vi "AddError__slk_mt.vi"(8 "error in (no error)":errorcluster, 10 "vi name":string, 11 "application reference":refnum<vi>) -> (0 "error out":errorcluster)   [LabVIEW 2013, in "Lazyboots Menu Tool.lvlib"]
doc: "This VI is the core of <b>Add Error</b> function, and will be called by corresponding menu launcher."
uses:
  Library/Lazyboots Menu Tool.lvlib
  <vilib>/Utility/config.llb/NI_LVConfig.lvlib
  Private/AddError/TypeDef/TypeDef_AddErrorState__slk_mt.ctl
  <vilib>/Utility/miscctls.llb/LVPositionTypeDef.ctl
panel:
  # "AddError__slk_mt.vi\nThis VI is the core of <b>Add Error</b> function, and will be called by corresponding menu launcher.\n\nNOTICE -- YOU MUST LEAVE THIS NOTICE IN PLACE.\n\nCopyright (c) 2011, LIANG LIU Shawn.Liu.cn@gmail.com\nAll rights reserved.\n\nRedistribution and use in source and binary forms, with or without modification, are permitted provided that the following conditions are met:\n-Redistributions of source code must retain the above copyright notice, this list of conditions and the following disclaimer.\n-Redistributions in binary form must reproduce the above copyright notice, this list of conditions and the following disclaimer in the documentation and/or other materials provided with the distribution.\n-Neither the name of the eLp nor the names of its contributors may be used to endorse or promote products derived from this software without specific prior written permission.\n\nTHIS SOFTWARE IS PROVIDED BY THE COPYRIGHT HOLDERS AND CONTRIBUTORS \"AS IS\" AND ANY EXPRESS OR IMPLIED WARRANTIES, INCLUDING, BUT NOT LIMITED TO, THE IMPLIED WARRANTIES OF MERCHANTABILITY AND FITNESS FOR A PARTICULAR PURPOSE ARE DISCLAIMED. IN NO EVENT SHALL THE COPYRIGHT HOLDER OR CONTRIBUTORS BE LIABLE FOR ANY DIRECT, INDIRECT, INCIDENTAL, SPECIAL, EXEMPLARY, OR CONSEQUENTIAL DAMAGES (INCLUDING, BUT NOT LIMITED TO, PROCUREMENT OF SUBSTITUTE GOODS OR SERVICES; LOSS OF USE, DATA, OR PROFITS; OR BUSINESS INTERRUPTION) HOWEVER CAUSED AND ON ANY THEORY OF LIABILITY, WHETHER IN CONTRACT, STRICT LIABILITY, OR TORT (INCLUDING NEGLIGENCE OR OTHERWISE) ARISING IN ANY WAY OUT OF THE USE OF THIS SOFTWARE, EVEN IF ADVISED OF THE POSSIBILITY OF SUCH DAMAGE."
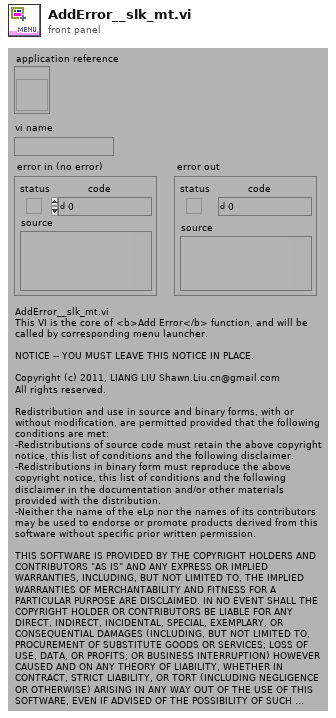
[diagram p1: front panel]
types:
  T1 = typedef "LVPositionTypeDef.ctl" = cluster{"Left":i32, "Top":i32}
  T2 = typedef "Lazyboots Menu Tool.lvlib/TypeDef_AddErrorState__slk_mt.ctl" = enum16{"Read Configure", "Get Menu Launch VI", "Get GObject Rectangle", "Calculate Error In Left Position", "Calculate Error In Top Position", "Undo.Start", "Add Error In", "Calculate Error Out Left Position", "Add Error Out", "Wire to Connector?", "Wire to Connector", "Undo.End/Fail", "End"}
  T3 = typedef "NI_LVConfig.lvlib/Config Data RefNum.ctl" = refnum<k1>
  T4 = typedef "Lazyboots Menu Tool.lvlib/TypeDef_AddErrorConfigure__slk_mt.ctl" = cluster{"Frame Width":u32, "Snap to Grid":bool, "FP Grid Size":u32, "Wire to Connector":bool, "Connector Pattern":u32, "Control Style":string, "Error Style":string}
  T5 = typedef "LVPointTypeDef.ctl" = cluster{"Horizontal":i16, "Vertical":i16}
  T6 = cluster{"left":i16, "top":i16, "right":i16, "bottom":i16}
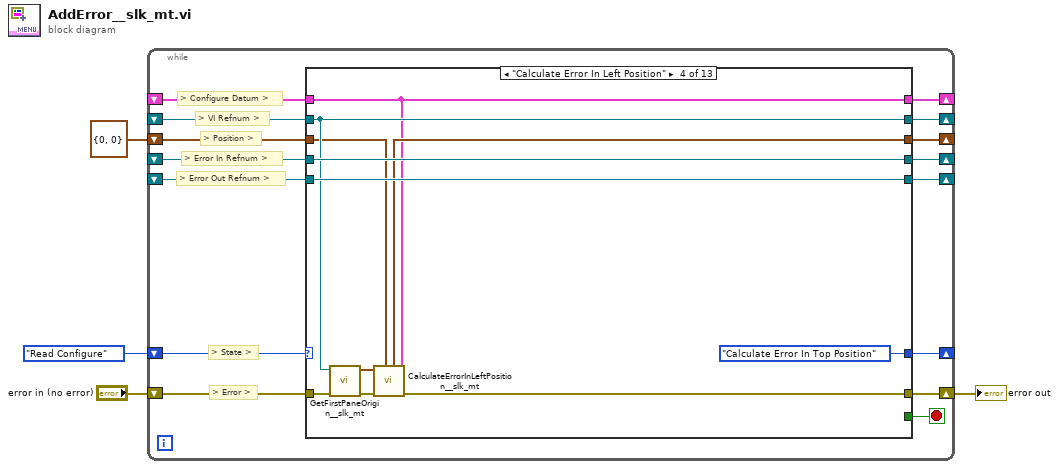
[diagram p0: block diagram]
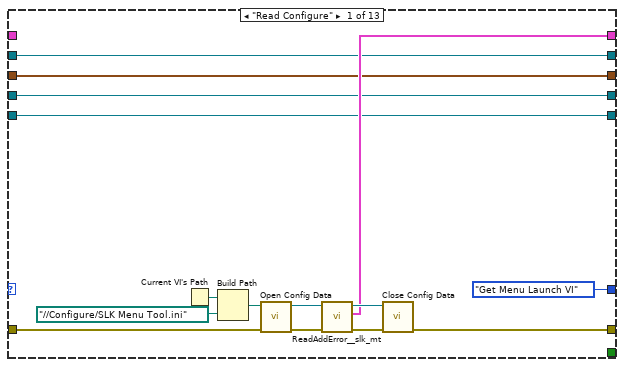
[diagram p2: hidden frame]
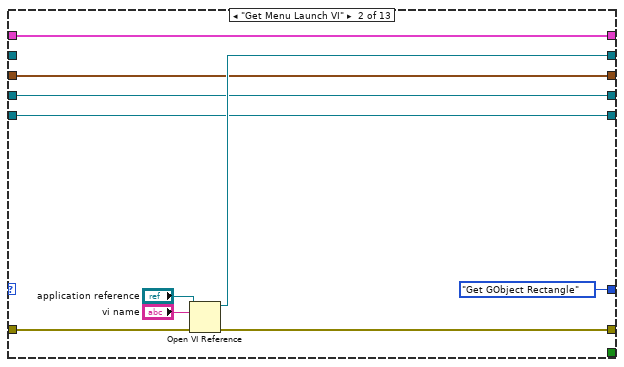
[diagram p3: hidden frame]
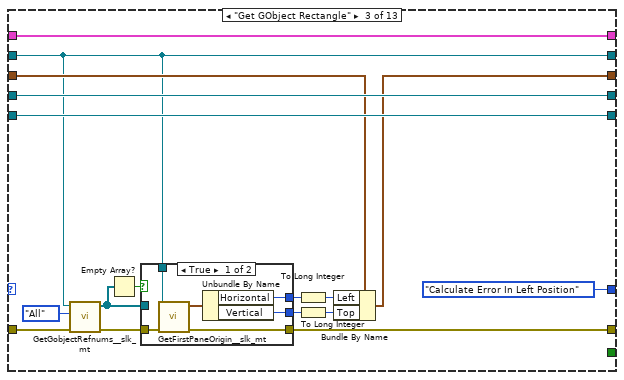
[diagram p4: hidden frame]
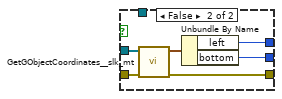
[diagram p5: hidden frame]
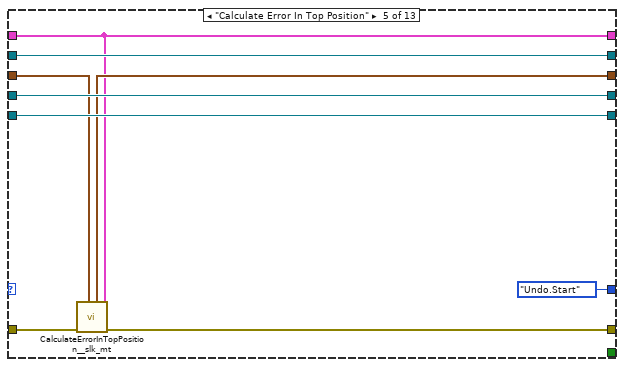
[diagram p6: hidden frame]
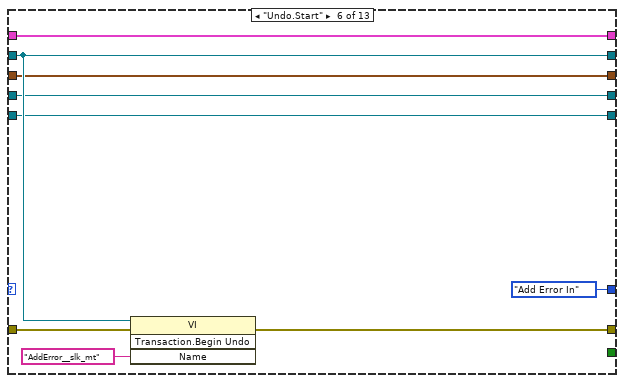
[diagram p7: hidden frame]
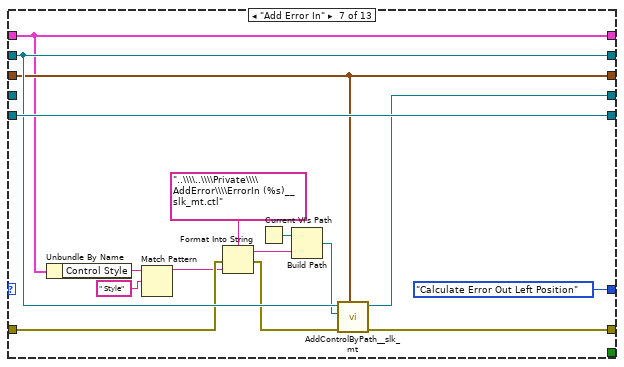
[diagram p8: hidden frame]
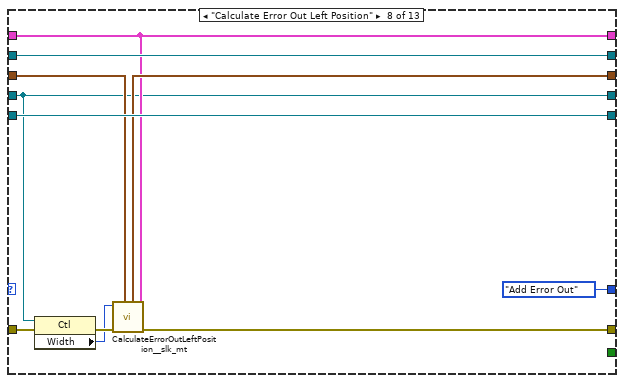
[diagram p9: hidden frame]
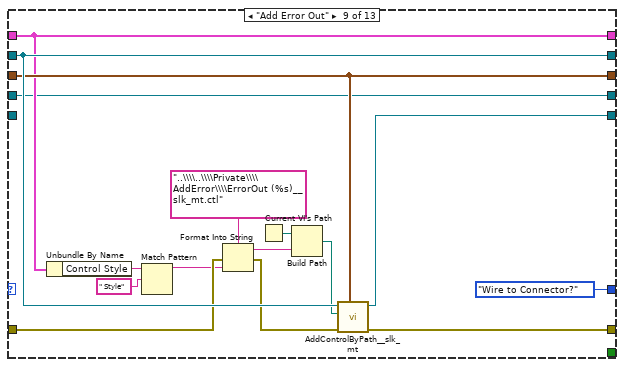
[diagram p10: hidden frame]
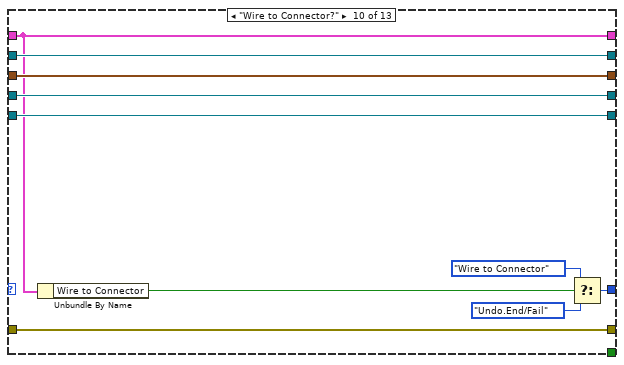
[diagram p11: hidden frame]
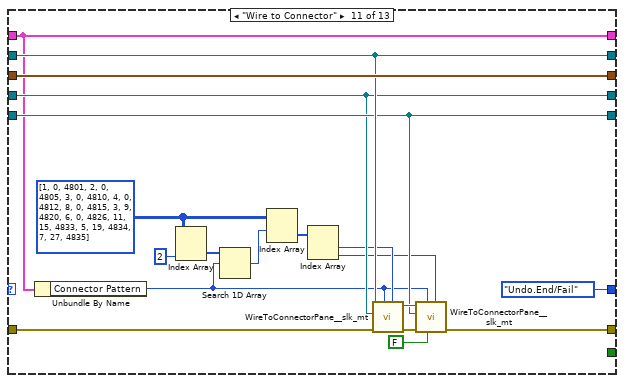
[diagram p12: hidden frame]
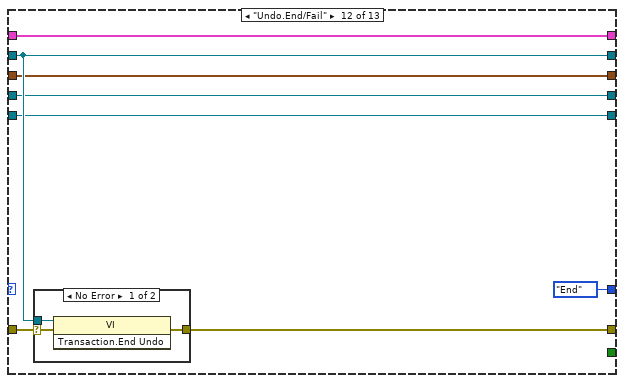
[diagram p13: hidden frame]
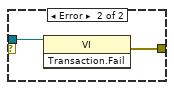
[diagram p14: hidden frame]
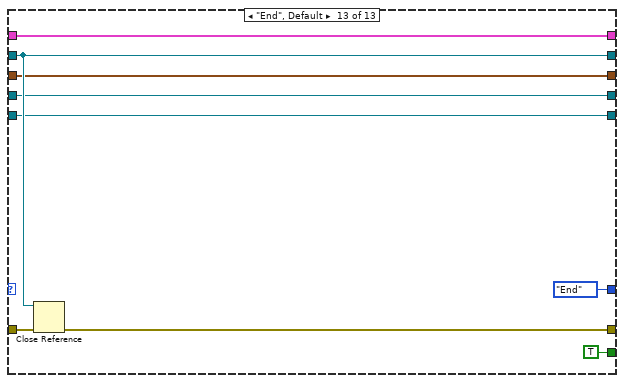
[diagram p15: hidden frame]
diagram:
  n1 = while {
    shift-right: [w16] -> _
    shift-left: TypeDef_AddErrorState__slk_mt."Read Configure" ("State") -> [w19]
    shift-right: [w17] -> w1
    shift-left: "error in (no error)" -> [w18]
    shift-right: [w14] -> _
    shift-left: _ -> [w15]
    shift-right: [w12] -> _
    shift-left: _ -> [w13]
    shift-right: [w7] -> _
    shift-left: T1 {"Left"=0, "Top"=0} ("Position") -> [w10]
    shift-right: [w6] -> _
    shift-left: _ -> [w9]
    shift-right: [w5] -> _
    shift-left: _ -> [w8]
    stop <- w11 stop-if-true
    # "> Error Out Refnum >"
    # "> Error In Refnum >"
    # "> Position >"
    # "> VI Refnum >"
    # "> Configure Datum >"
    # "> Error >"
    # "> State >"
    n2 = case shown="\"Calculate Error In Left Position\"" w19 {
      tunnel: w18 -> [w28 w44 w60 w82 w85 w101 w106 w122 w133 w155 w167 w180 w191]
      tunnel: [w26 w42 w56 w81 w91 w100 w116 w128 w144 w155 w166 w179 w193] -> w17
      tunnel: [TypeDef_AddErrorState__slk_mt."Get Menu Launch VI" ("State") TypeDef_AddErrorState__slk_mt."Get GObject Rectangle" ("State") TypeDef_AddErrorState__slk_mt."Calculate Error In Left Position" ("State") TypeDef_AddErrorState__slk_mt."Calculate Error In Top Position" ("State") TypeDef_AddErrorState__slk_mt."Undo.Start" ("State") TypeDef_AddErrorState__slk_mt."Add Error In" ("State") TypeDef_AddErrorState__slk_mt."Calculate Error Out Left Position" ("State") TypeDef_AddErrorState__slk_mt."Add Error Out" ("State") TypeDef_AddErrorState__slk_mt."Wire to Connector?" ("State") w152 TypeDef_AddErrorState__slk_mt."Undo.End/Fail" ("State") TypeDef_AddErrorState__slk_mt."End" ("State") TypeDef_AddErrorState__slk_mt."End" ("State")] -> w16
      tunnel: w15 -> [_ w41 w61 w75 w87 w102 w112 w124 w141 w147 w164 w182 w196]
      tunnel: [w24 w41 w61 w75 w87 w102 w112 w124 w141 w147 w164 w182 w196] -> w14
      tunnel: w13 -> [w23 _ w45 w79 w90 w99 w115 w127 w143 w151 w172 w178 w192]
      tunnel: [w23 w40 w45 w79 w90 w99 w115 w127 w143 w151 w172 w178 w192] -> w12
      tunnel: [_ _ _ _ _ _ _ _ _ _ _ _ TRUE] -> w11
      tunnel: w10 -> [w22 w38 w50 w77 w89 w96 w114 w126 w142 w150 w174 w177 w190]
      tunnel: w9 -> [w21 w37 w52 w84 w93 w95 _ w120 w135 w149 w169 w176 w189]
      tunnel: w8 -> [w20 w36 w51 w83 w92 w94 w117 w129 _ w148 w170 w175 w188]
      tunnel: [w22 w38 w49 w76 w88 w96 w114 w125 w142 w150 w174 w177 w190] -> w7
      tunnel: [w21 w37 w52 w84 w93 w95 w113 w120 w135 w149 w169 w176 w189] -> w6
      tunnel: [w20 w36 w51 w83 w92 w94 w117 w129 w134 w148 w170 w175 w188] -> w5
      frame "Read Configure" {
        n3 = Current VI's Path() -> (path=w30:path)
        n4 = Build Path(base path=w30, name or relative path=path "../../Configure/SLK Menu Tool.ini") -> (appended path=w29:path)
        n5 = call <vilib>:"Open Config Data.vi"("error in (no error)"=w28, "configuration file path"=w29) -> ("error out"=w33:errorcluster, "refnum"=w34:T3)  [unwired: 7 in, 1 out]
        n6 = call "ReadAddError__slk_mt.vi"("error in (no error)"=w33, "refnum in"=w34) -> ("error out"=w32:errorcluster, "add error configure"=w24:T4, "refnum out"=w31:T3)  [unwired: 7 in]
        n7 = call <vilib>:"Close Config Data.vi"("error in (no error)"=w32, "refnum"=w31) -> ("error out"=w26:errorcluster)  [unwired: 8 in, 1 out]
      }
      frame "Get Menu Launch VI" {
        n8 = Open VI Reference(application reference (local)="application reference", vi path="vi name", error in (no error)=w44) -> (vi reference=w40:refnum<vi>, error out=w42:errorcluster)  [unwired: 3 out]
      }
      frame "Get GObject Rectangle" {
        n9 = call "GetGobjectRefnums__slk_mt.vi"("error in (no error)"=w60, "from (Selected)"=enum16{"All", "Selected"}."All", "vi refnum in"=w45) -> ("error out"=w59:errorcluster, "generic objects refnums out"=w57:refnum<vi>[])  [unwired: 7 in]
        n10 = Empty Array?(array=w57) -> (empty?=w46:bool)
        n11 = case shown="True" w46 {
          tunnel: w59 -> [w67 w73]
          tunnel: w57 -> [_ w72]
          tunnel: [w66 w71] -> w56
          tunnel: [w64 w69] -> w54
          tunnel: [w63 w68] -> w53
          tunnel: w45 -> [w62 _]
          frame True {
            n12 = call "GetFirstPaneOrigin__slk_mt.vi"("error in (no error)"=w67, "vi refnum in"=w62) -> ("error out"=w66:errorcluster, "origin"=w65:T5)  [unwired: 8 in]
            n13 = Unbundle By Name(w65) -> ("Horizontal"=w64:i16, "Vertical"=w63:i16)
          }
          frame False {
            n14 = call "GetGObjectCoordinates__slk_mt.vi"("error in (no error)"=w73, "generic objects refnums in"=w72) -> ("error out"=w71:errorcluster, "rectangle"=w70:T6)  [unwired: 6 in, 2 out]
            n15 = Unbundle By Name(w70) -> ("left"=w69:i16, "bottom"=w68:i16)
          }
        }
        n16 = To Long Integer(number=w54) -> (32bit integer=w48:i32)
        n17 = To Long Integer(number=w53) -> (32bit integer=w47:i32)
        n18 = Bundle By Name(cluster=w50, "Left"=w48, "Top"=w47) -> (w49:T1)
      }
      frame "Calculate Error In Left Position" {
        n19 = call "GetFirstPaneOrigin__slk_mt.vi"("error in (no error)"=w82, "vi refnum in"=w79) -> ("error out"=w80:errorcluster, "origin"=w78:T5)  [unwired: 8 in]
        n20 = call "CalculateErrorInLeftPosition__slk_mt.vi"("add error configure"=w75, "position in"=w77, "error in (no error)"=w80, "origin (0,0)"=w78) -> ("error out"=w81:errorcluster, "position out"=w76:T1)  [unwired: 6 in]
      }
      frame "Calculate Error In Top Position" {
        n21 = call "CalculateErrorInTopPosition__slk_mt.vi"("add error configure"=w87, "position in"=w89, "error in (no error)"=w85) -> ("error out"=w91:errorcluster, "position out"=w88:T1)  [unwired: 7 in]
      }
      frame "Undo.Start" {
        n22 = invoke class="VI" method="Transaction.Begin Undo"(reference=w99, error in=w101, "Name"="AddError__slk_mt") -> (error out=w100:errorcluster)  [unwired: 1 in, 3 out]
      }
      frame "Add Error In" {
        n23 = Unbundle By Name(w112) -> ("Control Style"=w104:string)
        n24 = Match Pattern(string=w104, regular expression=" Style" ("format string")) -> (before substring=w105:string)  [unwired: 1 in, 3 out]
        n25 = Format Into String(format string="..\\\\..\\\\Private\\\\AddError\\\\ErrorIn (%s)__slk_mt.ctl", error in=w106, w105) -> (resulting string=w110:string, error out=w107:errorcluster)  [unwired: 1 in]
        n26 = Current VI's Path() -> (path=w111:path)
        n27 = Build Path(base path=w111, name or relative path=w110) -> (appended path=w109:path)
        n28 = call "AddControlByPath__slk_mt.vi"("position (0,0)"=w114, "error in (no error)"=w107, "path"=w109, "owner vi refnum in"=w115) -> ("error out"=w116:errorcluster, "control refnum out"=w113:refnum<vi>)  [unwired: 6 in]
      }
      frame "Calculate Error Out Left Position" {
        n29 = property class="Ctl"(reference=w120, error in=w122) -> (error out=w121:errorcluster, "Width"=w119:u32)  [unwired: 1 out]
        n30 = call "CalculateErrorOutLeftPosition__slk_mt.vi"("add error configure"=w124, "position in"=w126, "error in (no error)"=w121, "\"error in\" width"=w119) -> ("error out"=w128:errorcluster, "position out"=w125:T1)  [unwired: 6 in]
      }
      frame "Add Error Out" {
        n31 = Unbundle By Name(w141) -> ("Control Style"=w130:string)
        n32 = Match Pattern(string=w130, regular expression=" Style" ("format string")) -> (before substring=w132:string)  [unwired: 1 in, 3 out]
        n33 = Format Into String(format string="..\\\\..\\\\Private\\\\AddError\\\\ErrorOut (%s)__slk_mt.ctl", error in=w133, w132) -> (resulting string=w139:string, error out=w136:errorcluster)  [unwired: 1 in]
        n34 = Current VI's Path() -> (path=w140:path)
        n35 = Build Path(base path=w140, name or relative path=w139) -> (appended path=w138:path)
        n36 = call "AddControlByPath__slk_mt.vi"("position (0,0)"=w142, "error in (no error)"=w136, "path"=w138, "owner vi refnum in"=w143) -> ("error out"=w144:errorcluster, "control refnum out"=w134:refnum<vi>)  [unwired: 6 in]
      }
      frame "Wire to Connector?" {
        n37 = Unbundle By Name(w147) -> ("Wire to Connector"=w146:bool)
        n38 = Select(t=TypeDef_AddErrorState__slk_mt."Wire to Connector" ("State"), s=w146, f=TypeDef_AddErrorState__slk_mt."Undo.End/Fail" ("State")) -> (s? t:f=w152:T2)
      }
      frame "Wire to Connector" {
        w161 = u32[][] [[1, 0, 4801], [2, 0, 4805], [3, 0, 4810], [4, 0, 4812], [8, 0, 4815], [3, 9, 4820], [6, 0, 4826], [11, 15, 4833], [5, 19, 4834], [7, 27, 4835]]
        n39 = Unbundle By Name(w164) -> ("Connector Pattern"=w156:u32)
        n40 = Index Array(array=w161, index (col)=2 ("disabled index (col)")) -> (element=w162:u32[])  [unwired: 1 in]
        n41 = Search 1D Array(1D array=w162, element=w156) -> (index of element=w160:i32)  [unwired: 1 in]
        n42 = Index Array(array=w161, index (row)=w160) -> (element=w159:u32[])  [unwired: 1 in]
        n43 = Index Array(array=w159) -> (element #1=w158:u32, element #2=w157:u32)  [unwired: 2 in]
        n44 = call "WireToConnectorPane__slk_mt.vi"("terminal index"=w158, "pattern (no change: 0)"=w156, "error in (no error)"=w167, "control refnum in"=w169, "vi refnum in"=w172) -> ("error out"=w168:errorcluster, "duplicated vi refnum out"=w171:refnum<vi>)  [unwired: 5 in]
        n45 = call "WireToConnectorPane__slk_mt.vi"("terminal index"=w157, "icon visible? (T)"=FALSE, "pattern (no change: 0)"=w156, "error in (no error)"=w168, "control refnum in"=w170, "vi refnum in"=w171) -> ("error out"=w166:errorcluster)  [unwired: 4 in, 1 out]
      }
      frame "Undo.End/Fail" {
        n46 = case shown="No Error" w180 {
          selector: w180 -> [w184 _]
          tunnel: w178 -> [w185 w187]
          tunnel: [w183 w186] -> w179
          frame No Error {
            n47 = invoke class="VI" method="Transaction.End Undo"(reference=w185, error in=w184) -> (error out=w183:errorcluster)  [unwired: 1 in, 2 out]
          }
          frame Error {
            n48 = invoke class="VI" method="Transaction.Fail"(reference=w187) -> (error out=w186:errorcluster)  [unwired: 2 in, 2 out]
          }
        }
      }
      frame "End", Default {
        n49 = Close Reference(reference=w192, error in (no error)=w191) -> (error out=w193:errorcluster)
      }
    }
  }
  "error out" <- w1
